vi "Filter Shortcut Menu Activation Event.vi"(8 "error in (no error)":errorcluster, 10 "ShortcutMenuActivationMsg":refnum<class "ShortcutMenuActivationMsg.lvclass">, 11 "Test Executive Builder Event Filter in":refnum<class "Test Executive Builder Event Filter.lvclass">) -> (0 "error out":errorcluster, 1 "Discard?":bool, 3 "Test Executive Builder Event Filter out":refnum<class "Test Executive Builder Event Filter.lvclass">)   [LabVIEW 2017, in "Test Executive Builder Event Filter.lvclass"]
uses:
  Test Executive Builder Event Filter.lvclass
  <vilib>/gpm_packages/@cs/mva-viewable/Source/ActorEvents/IEventAggregator Messages/ShortcutMenuActivationMsg/ShortcutMenuActivationMsg.lvclass
  Test Executive Builder View Messages/Populate Menu Msg/Populate Menu Msg.lvclass
  <vilib>/gpm_packages/@cs/actor-framework-messages/Source/RoundTripMessage/RoundTripMessage.lvclass
  C:/Users/jonmc/Documents/Git/Test Executive Builder/gpm_packages/@cs/actor-framework-messages/Source/RoundTripMessage/RoundTripMessage.lvclass
panel:
  # "No additional\nEvent Data"
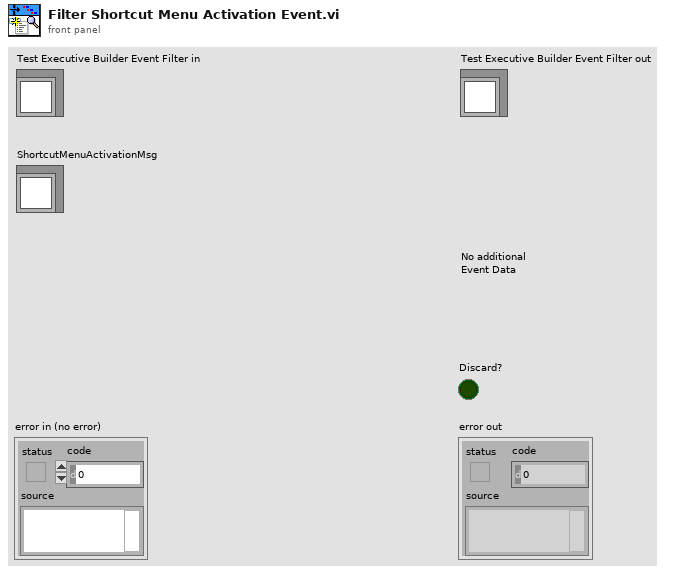
[diagram p1: front panel]
types:
  T1 = typedef "LVPoint32TypeDef.ctl" = cluster{"Horizontal":i32, "Vertical":i32}
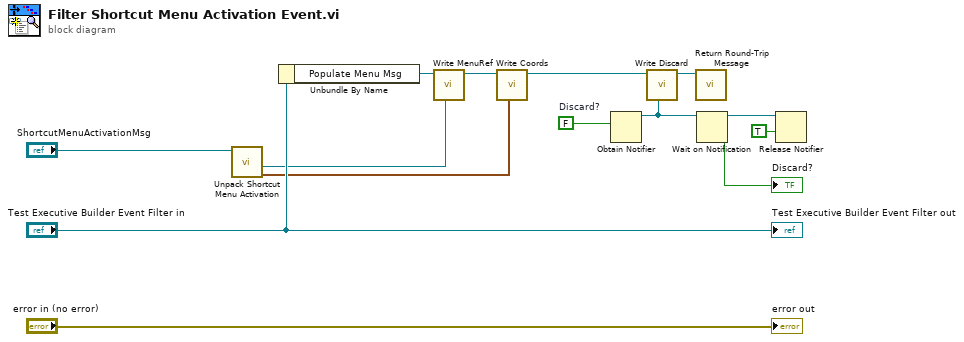
[diagram p0: block diagram]
diagram:
  w12 = FALSE  # Discard?
  n1 = call <vilib>:"Unpack Shortcut Menu Activation.vi"("ShortcutMenuActivationMsg"="ShortcutMenuActivationMsg") -> ("Coords"=w3:T1, "MenuRef"=w6:refnum<k9>)  [unwired: 5 in, 4 out]
  n2 = Unbundle By Name("Test Executive Builder Event Filter in") -> ("Populate Menu Msg"=w7:refnum<class "Populate Menu Msg.lvclass">)
  n3 = call "Write MenuRef.vi"("MenuRef"=w6, "Populate Menu Msg in"=w7) -> ("Populate Menu Msg out"=w5:refnum<class "Populate Menu Msg.lvclass">)  [unwired: 9 in]
  n4 = call "Write Coords.vi"("Coordinates"=w3, "Populate Menu Msg in"=w5) -> ("Populate Menu Msg out"=w4:refnum<class "Populate Menu Msg.lvclass">)  [unwired: 9 in]
  n5 = Obtain Notifier(notification data type=w12) -> (notifier out=w10:refnum<notifier>)  [unwired: 3 in, 2 out]
  n6 = call "Write Discard.vi"("Discard?"=w10, "Populate Menu Msg in"=w4) -> ("Populate Menu Msg out"=w1:refnum<class "Populate Menu Msg.lvclass">)  [unwired: 9 in]
  n7 = call <vilib>:"Return Round-Trip Message.vi"("RoundTripMessage In"=w1) -> ()  [unwired: 10 in, 1 out]
  n8 = Wait on Notification(notifier=w10) -> (notifier out=w8:refnum<notifier>, notification=→"Discard?":bool)  [unwired: 3 in, 2 out]
  n9 = Release Notifier(notifier=w8, force destroy? (F)=TRUE) -> ()  [unwired: 1 in, 3 out]
  "error out" <- "error in (no error)"
  "Test Executive Builder Event Filter out" <- "Test Executive Builder Event Filter in"
